vi "niFPGA SQRT Integer (32 bit) - Rounded.vi"(4 "x [U32]":u32) -> (1 "sqrt (x) [U16]":u16)   [LabVIEW 2017]
doc: "Iteratively computes the rounded integer square root of an unsigned 32-bit input using a binary restoring square root extraction algorithm. The rounding mode is round to nearest (+Inf), in which one extra bit is computed to determine whether to round up or down.\n\nNOTE: Input values must be less than 65535.5^2 (ie, less than or equal to 4294901760 or xFFFF0000) in order to avoid overflowing the output U16 integer. Overflow will result in an output of zero."
uses:
  <vilib>/Platform/TimedLoop/XDataNode/timing_clust.ctl
  <vilib>/Platform/TimedLoop/XDataNode/nitl_modes.ctl
  <vilib>/Platform/TimedLoop/XDataNode/wakeup.ctl
  <vilib>/Platform/TimedLoop/XDataNode/XDataNode.xnode
  <vilib>/Platform/TimedLoop/XDataNode/XDNodeRunTimeDep.lvlib
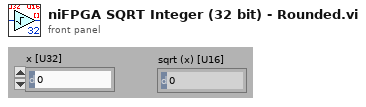
[diagram p1: front panel]
types:
  T1 = typedef "XDNodeRunTimeDep.lvlib/timing_clust.ctl" = cluster{"Expected End [f-1]":u64, "Actual End [f-1]":u64, "Finished Late? [f-1]":bool, "Expected End [i-1]":u64, "Actual End [i-1]":u64, "Finished Late? [i-1]":bool, "Expected Start [i]":u64, "Actual Start [i]":u64, "Expected Start [f]":u64, "Actual Start [f]":u64, "Source Name":string, "Structure Name":string, "Period":i64, "Deadline":i64, "Offset":i64, "Start":i64, "Priority":i32, "Timeout":i32, "Mode":T2, "Wakeup Reason":T3, "Error":errorcluster, "Source Type":string, "Secondary Source Type":string, "Global End Time":u64, "Global Start Time":u64, "Frame Duration":u64, "Iteration Duration":u64, "Assigned CPU":i32, "I/O Scan Engine Mode":u32}
  T2 = typedef "XDNodeRunTimeDep.lvlib/nitl_modes.ctl" = enum32{"No Change", "Process missed periods, maintain original phase", "Discard missed periods, maintain original phase", "Process missed periods, ignore original phase", "Discard missed periods, ignore original phase"}
  T3 = typedef "XDNodeRunTimeDep.lvlib/wakeup.ctl" = enum32{"Normal", "Aborted", "Asynchronous wakeup", "Timing source error", "Timed loop error", "Timeout"}
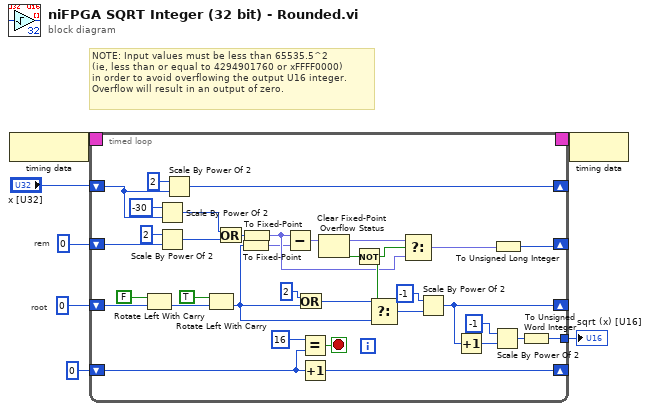
[diagram p0: block diagram]
diagram:
  # "NOTE: Input values must be less than 65535.5^2 \n(ie, less than or equal to 4294901760 or xFFFF0000) \nin order to avoid overflowing the output U16 integer. \nOverflow will result in an output of zero."
  # "rem"
  # "root"
  n1 = node-c288() -> (w4:T1)
  n2 = timed-loop {
    timing-out: [_] -> w5
    timing: w4 -> [_]
    shift-left: u32 0 ("x [U32.2]") -> [w35]
    shift-right: [w12] -> _
    shift-left: u32 0 ("x [U32.2]") -> [w42]
    shift-right: [w17] -> _
    shift-left: "x [U32]" -> [w39]
    shift-right: [w36] -> _
    tunnel: [w15] -> w2
    shift-right: [w19] -> _
    shift-left: u8 0 -> [w20]
    stop <- w18 stop-if-true
    n3 = Rotate Left With Carry(2:w42, 3:FALSE ("carry")) -> (0:w33:u32)  [unwired: 1 out]
    n4 = Scale By Power Of 2(n=i8 -30, x=w39) -> (x*2^n=w11:u32)
    n5 = Scale By Power Of 2(n=i8 2, x=w35) -> (x*2^n=w10:u32)
    n6 = Scale By Power Of 2(n=i8 2, x=w39) -> (x*2^n=w36:u32)
    n7 = Rotate Left With Carry(2:w33, 3:TRUE ("carry")) -> (0:w28:u32)  [unwired: 1 out]
    n8 = Or(x=w11, y=w10) -> (x .or. y?=w25:u32)
    n9 = To Fixed-Point(number=w28) -> (fixed-point=w9:fxp<+,32,32>)  [unwired: 1 out]
    n10 = To Fixed-Point(number=w25) -> (fixed-point=w13:fxp<+,32,32>)  [unwired: 1 out]
    n11 = Subtract(x=w13, y=w9) -> (x-y=w26:fxp<+,32,32>)
    n12 = Or(x=u32 2, y=w28) -> (x .or. y?=w30:u32)
    n13 = Equal?(x=u8 16, y=w20) -> (x = y?=w18:bool)
    n14 = Increment(x=w20) -> (x+1=w19:u8)
    n15 = Clear Fixed-Point Overflow Status(3:w26) -> (0:w8:bool, 1:w14:fxp<+,32,32>)
    n16 = Not(x=w8) -> (.not. x?=w27:bool)
    n17 = Select(t=w30, s=w27, f=w28) -> (s? t:f=w29:u32)
    n18 = Select(t=w14, s=w27, f=w13) -> (s? t:f=w24:fxp<+,32,32>)
    n19 = Scale By Power Of 2(n=-1, x=w29) -> (x*2^n=w17:u32)
    n20 = Increment(x=w17) -> (x+1=w16:u32)
    n21 = Scale By Power Of 2(n=-1, x=w16) -> (x*2^n=w23:u32)
    n22 = To Unsigned Long Integer(number=w24) -> (unsigned 32bit integer=w12:u32)
    n23 = To Unsigned Word Integer(number=w23) -> (unsigned 16bit integer=w15:u16)
  }
  "sqrt (x) [U16]" <- w2
  n24 = node-c288(w5) -> ()
